vi "Evaluate Part 2.vi"() -> ()   [LabVIEW 2021]
uses:
  e7b2fbfc-796b-4aad-801c-aef1de4c8643.vi
  Proto/Maze.lvclass
panel:
  out "Maze":string[][](array[string])
  out "size(s)":i32
  out "max value":u64
  in  "Input":string="#.#####################\n#.......#########...###\n#######.#########.#.###\n###.....#.>.>.###.#.###\n###v#####.#v#.###.#.###\n###.>...#.#.#.....#...#\n###v###.#.#.#########.#\n###...#.#.#.......#...#\n#####.#.#.#######.#.###\n#.....#.#.#.......#...#\n#.#####.#.#.#########v#\n#.#...#...#...###...>.#\n#.#.#v#######v###.###v#\n#...#.>.#...>.>.#.###.#\n#####v#.#.###v#.#.###.#\n#.....#...#...#.#.#...#\n#.#########.###.#.#.###\n#...###...#...#...#.###\n###.###.#.###v#####v###\n#...#...#.#.>.>.#.>.###\n#.###.###.#.###.#.#v###\n#.....###...###...#...#\n#####################.#"
  # "5664 too low\n5030 not right"
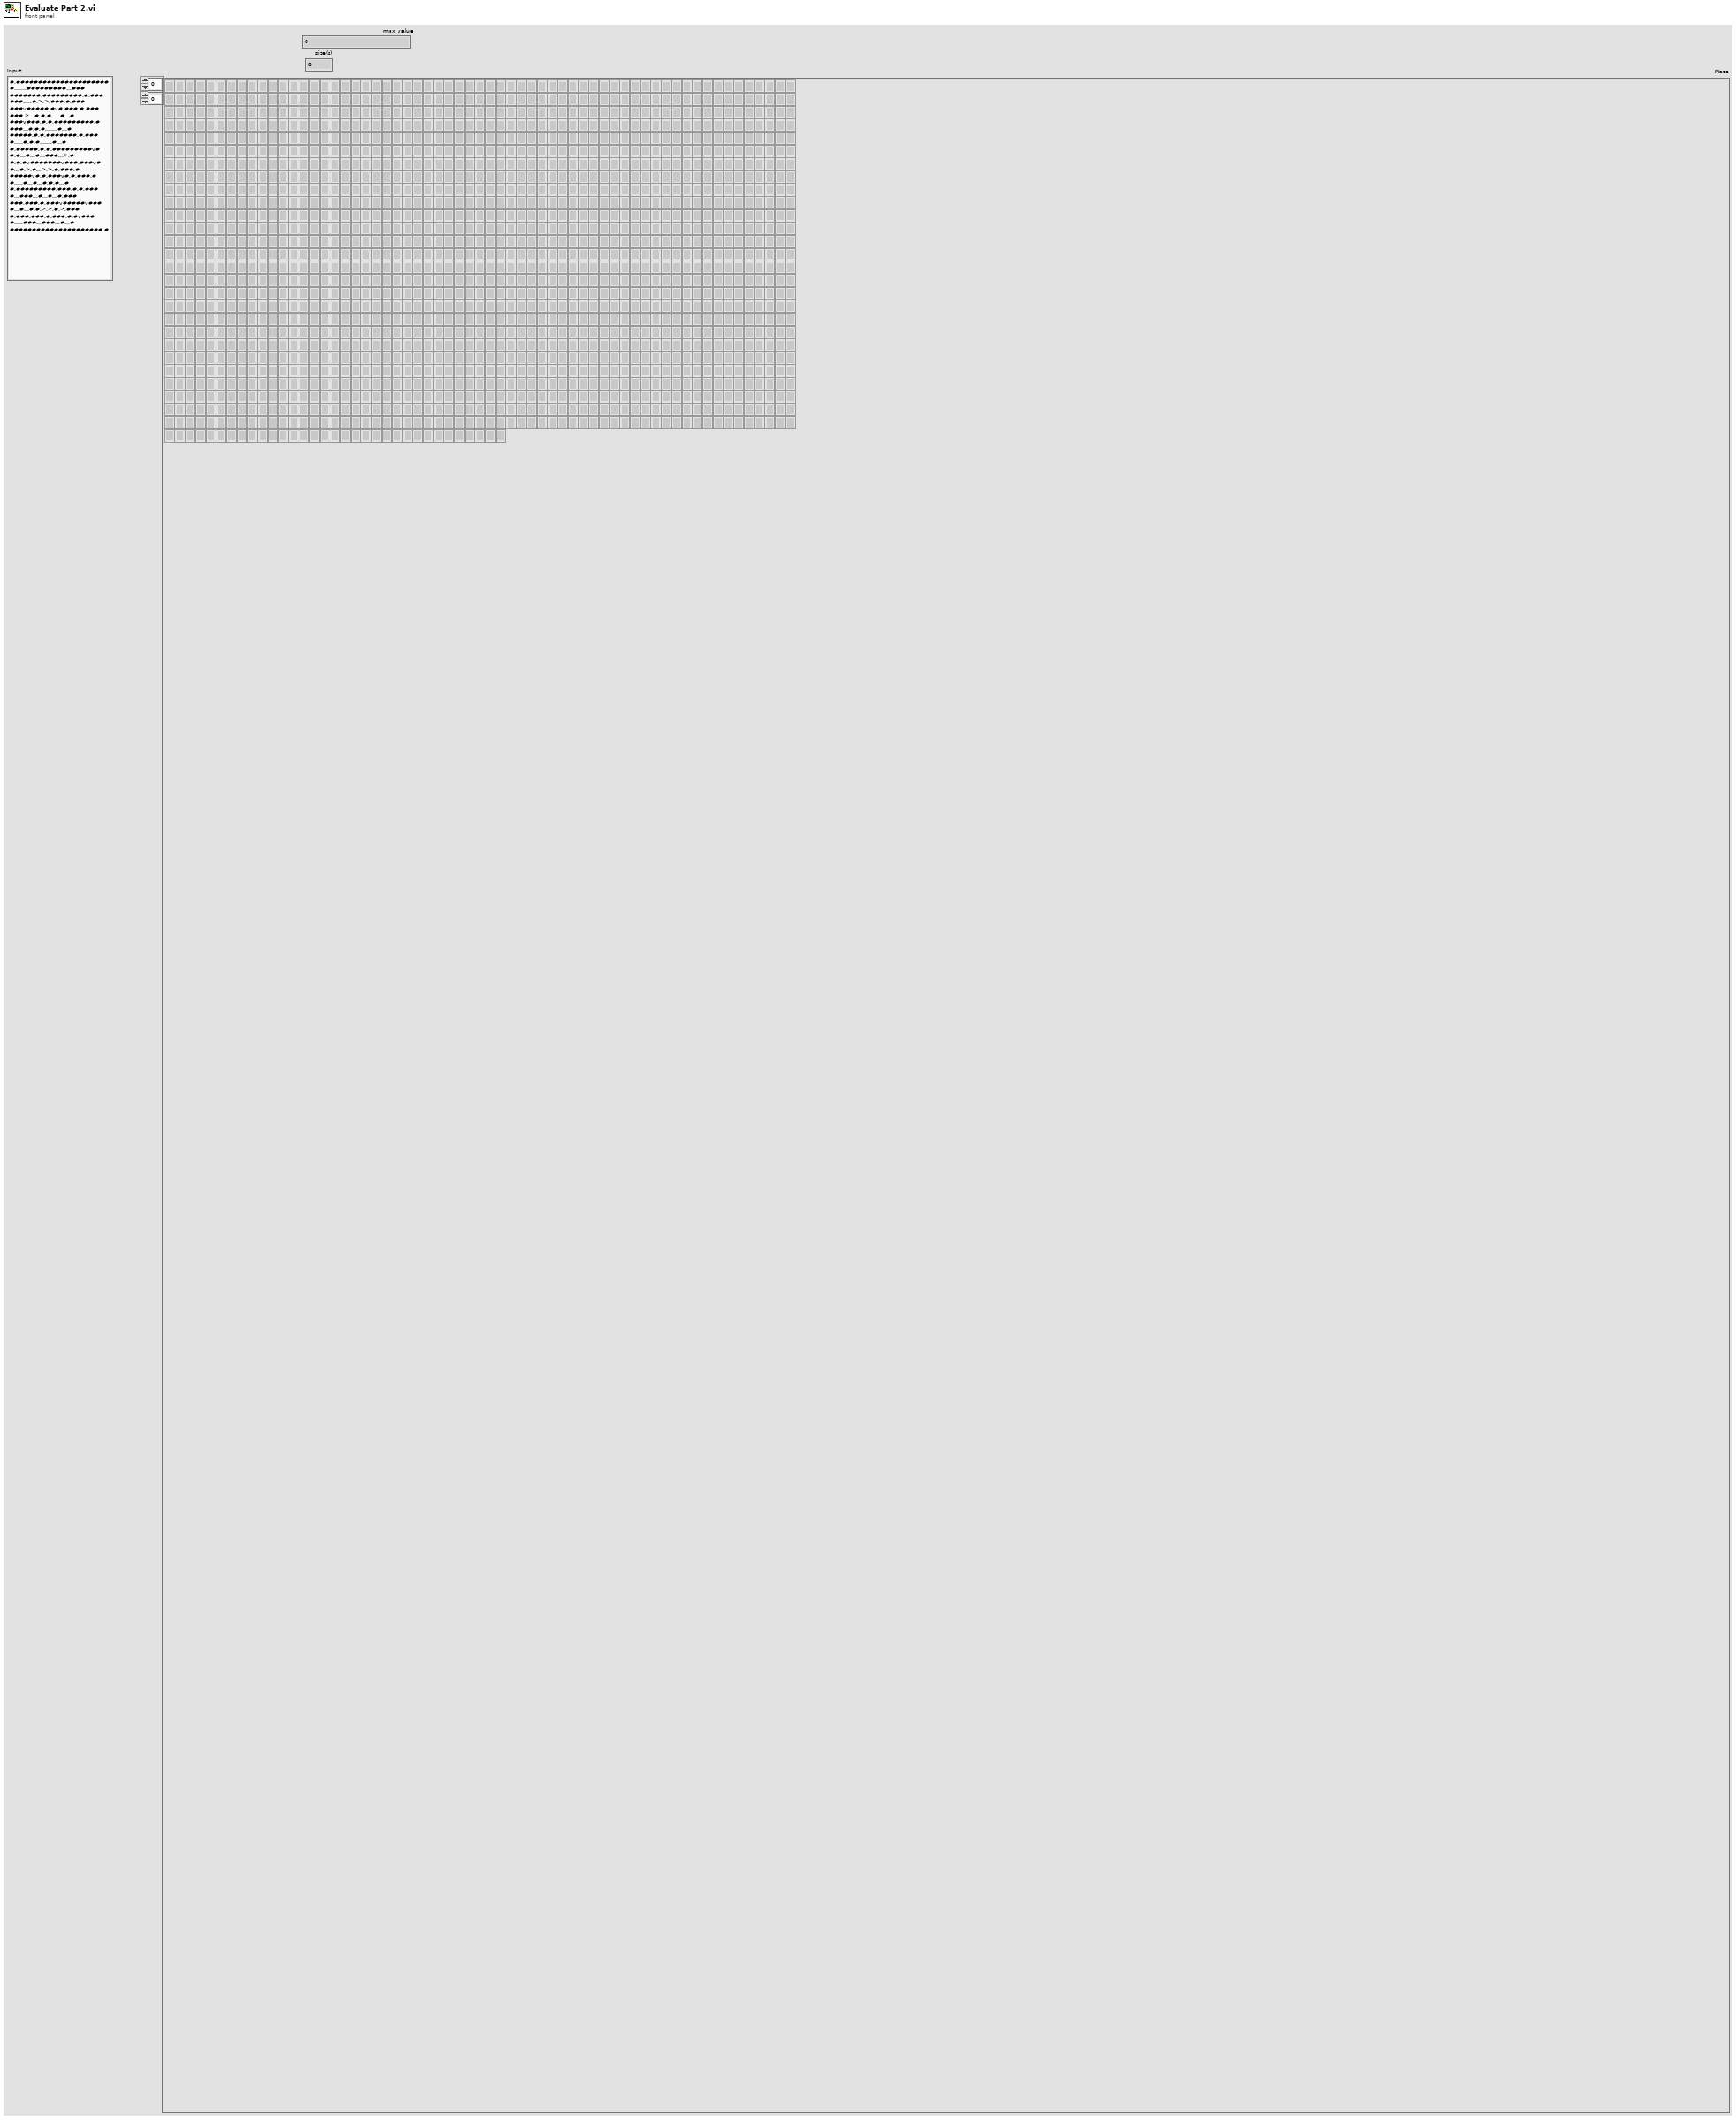
[diagram p1: front panel]
types:
  T1 = cluster{"row":i32, "col":i32, "Arriving from":enum16{"North", "South", "East", "West"}}
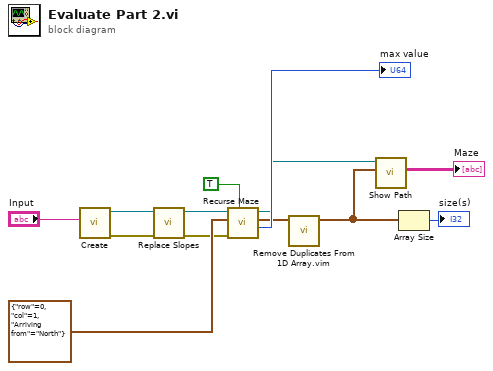
[diagram p0: block diagram]
diagram:
  n1 = call "Create.vi"("Input"="Input") -> ("error out"=w13:errorcluster, "Proto"=w8:refnum<class "Maze.lvclass">)  [unwired: 9 in]
  n2 = call "Replace Slopes.vi"("error in (no error)"=w13, "Maze in"=w8) -> ("error out"=w9:errorcluster, "Maze out"=w7:refnum<class "Maze.lvclass">)  [unwired: 8 in]
  n3 = call "Recurse Maze.vi"("Visit only once?"=TRUE, "error in (no error)"=w9, "Current Cell"=T1 {"row"=0, "col"=1, "Arriving from"=enum."North"} ("Possible Steps"), "Maze In"=w7) -> ("Step Count"=→"max value":i32, "Steps"=w4:cluster{"row":i32, "col":i32}[], "Maze Out"=w3:refnum<class "Maze.lvclass">)  [unwired: 4 in, 1 out]
  n4 = call "Remove Duplicates From 1D Array.vim"("array"=w4) -> ("array with duplicates removed"=w1:cluster{"row":i32, "col":i32}[])  [unwired: 10 in]
  n5 = call "Show Path.vi"("Steps"=w1, "Maze in"=w3) -> ("Maze"=→"Maze":string[][])  [unwired: 7 in, 2 out]
  n6 = Array Size(array=w1) -> (size(s)=→"size(s)":i32)
